vi "HP81110A Set Trigger Source.vi"(8 "error in (no error)":errorcluster, 10 "Trigger (Bit Period) Source (0:Immediate, via internal oscillator)":T1(ring), 11 "VISA session":refnum<visa-resource-name>) -> (0 "error out":errorcluster, 3 "dup VISA session":refnum<visa-resource-name>)   [LabVIEW 2009]
doc: "This VI sets the trigger (bit period) source. Options are: \n0 = Immediate (internal oscillator)\n1 = Internal PLL\n2 = Clock Input"
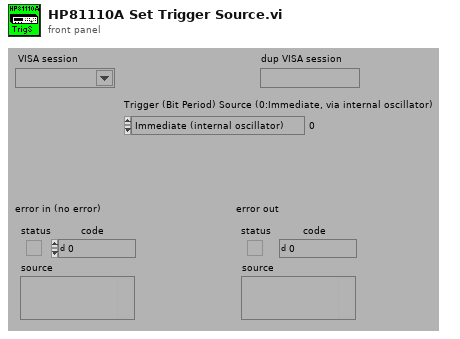
[diagram p1: front panel]
types:
  T1 = enum16{"Immediate (internal oscillator)", "Internal PLL", "Clock Input"}
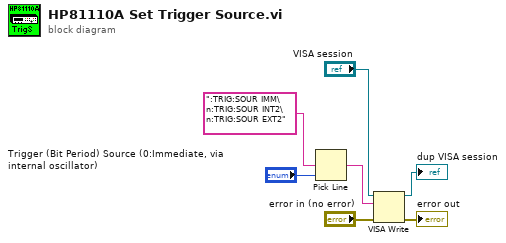
[diagram p0: block diagram]
diagram:
  n1 = Pick Line(multi-line string=":TRIG:SOUR IMM\n:TRIG:SOUR INT2\n:TRIG:SOUR EXT2", line index="Trigger (Bit Period) Source (0:Immediate, via internal oscillator)") -> (output string=w3:string)  [unwired: 1 out]
  n2 = VISA Write(VISA resource name="VISA session", write buffer=w3, error in (no error)="error in (no error)") -> (VISA resource name out=→"dup VISA session":refnum<visa-resource-name>, error out=→"error out":errorcluster)  [unwired: 1 out]
